vi "File Rollover.vi"() -> ()   [LabVIEW 2018]
uses:
  src/api/logger_class/Log Levels.ctl
  src/api/configuration/handlers/file_handler/File Handler.lvclass
  C:/Users/Colin/Documents/software_projects/labview/glog/src/api/extension/formatting_handler_interface/Formatting Handler.lvclass
  src/api/logger_class/Log (Parts).vi
  src/api/logger_class/Logger.lvclass
panel:
  in  "delete when done?":bool=TRUE
  out "error out":errorcluster
  out "2 files? (post-rollover)":bool
  out "1 file? (2nd)":bool
  out "1 file? (1st)":bool
  # "Locals"
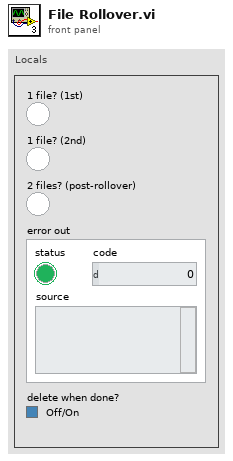
[diagram p1: front panel]
types:
  T1 = typedef "GLog.lvlib/Logger.lvclass/Log Levels.ctl" = enum16{"Trace", "Debug", "Info", "Warning", "Error", "Critical"}
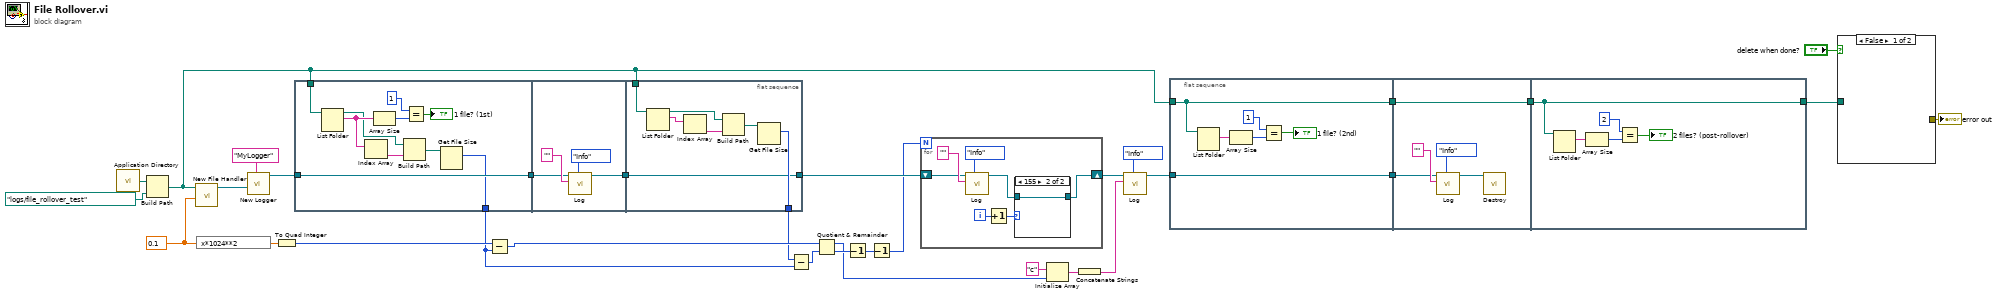
[diagram p0: block diagram]
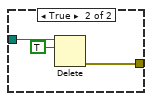
[diagram p3: hidden frame]
diagram:
  w26 = 0.1 ("rollover threshold [MB](50)")
  n1 = call <vilib>:"Application Directory.vi"() -> ("Application Directory"=w30:path)
  n2 = Build Path(base path=w30, name or relative path=path "logs/file_rollover_test") -> (appended path=w7:path)
  n3 = call "New File Handler.vi"("max file size [MB](50)"=w26, "log directory (<app dir>/logs)"=w7) -> ("file handler"=w31:refnum<class "File Handler.lvclass">)  [unwired: 9 in]
  n4 = expression code="x*1024**2"(w26) -> (w14:dbl)
  n5 = call "New Logger.vi"("name (\"Default\")"="MyLogger" ("name"), "log handler (file handler)"=w31) -> ("logger"=w9:refnum<class "Logger.lvclass">)  [unwired: 8 in, 1 out]
  n6 = To Quad Integer(1:w14) -> (0:w6:i64)
  n7 = flat-sequence {
    tunnel: w9 -> [w42]
    tunnel: [w42] -> w8
    tunnel: w7 -> [w35]
    tunnel: [w33] -> w4
    tunnel: [w43] -> w10
    tunnel: w8 -> [w44]
    tunnel: [w50] -> w3
    tunnel: w7 -> [w49]
    tunnel: [w48] -> w17
    tunnel: w10 -> [w48]
    frame #0 {
      n8 = List Folder(path=w35) -> (path out=w37:path, filenames=w39:string[])  [unwired: 3 in, 2 out]
      n9 = Index Array(array=w39) -> (element=w38:string)  [unwired: 1 in]
      n10 = Array Size(array=w39) -> (size(s)=w40:i32)
      n11 = Build Path(base path=w37, name or relative path=w38) -> (appended path=w36:path)
      n12 = Equal?(x=1, y=w40) -> (x = y?=→"1 file? (1st)":bool)
      n13 = Get File Size(file=w36) -> (size (in bytes)=w33:i64)  [unwired: 1 in, 2 out]
    }
    frame #1 {
      n14 = call-poly "Log.vi"("log level"=Log_Levels."Info" ("level"), "message"="", "logger in"=w44) -> ("logger out"=w43:refnum<class "Logger.lvclass">)  [unwired: 8 in]
    }
    frame #2 {
      n15 = List Folder(path=w49) -> (path out=w51:path, filenames=w53:string[])  [unwired: 3 in, 2 out]
      n16 = Index Array(array=w53) -> (element=w52:string)  [unwired: 1 in]
      n17 = Build Path(base path=w51, name or relative path=w52) -> (appended path=w47:path)
      n18 = Get File Size(file=w47) -> (size (in bytes)=w50:i64)  [unwired: 1 in, 2 out]
    }
  }
  n19 = Subtract(x=w6, y=w4) -> (x-y=w5:i64)
  n20 = Subtract(x=w3, y=w4) -> (x-y=w2:i64)
  n21 = Quotient & Remainder(x=w5, y=w2) -> (x-y*floor(x/y)=w19:i64, floor(x/y)=w25:i64)
  n22 = Decrement(x=w25) -> (x-1=w24:i64)
  n23 = Decrement(x=w24) -> (x-1=w16:i64)
  n24 = for {
    N: w16 -> [_]
    shift-right: [w55] -> w23
    shift-left: w17 -> [w57]
    i -> [w58]
    n25 = call-poly "Log.vi"("log level"=Log_Levels."Info" ("level"), "message"="", "logger in"=w57) -> ("logger out"=w56:refnum<class "Logger.lvclass">)  [unwired: 8 in]
    n26 = Increment(x=w58) -> (x+1=w54:i32)
    n27 = case shown="155" w54 {
      tunnel: w56 -> [w61 w62]
      tunnel: [w61 w62] -> w55
      frame Default {
      }
      frame 155 {
      }
    }
  }
  n28 = Initialize Array("c" ("message"), w19) -> (w21:string[])
  n29 = Concatenate Strings(w21) -> (w18:string)
  n30 = call-poly "Log.vi"("log level"=Log_Levels."Info" ("level"), "message"=w18, "logger in"=w23) -> ("logger out"=w12:refnum<class "Logger.lvclass">)  [unwired: 8 in]
  n31 = flat-sequence {
    tunnel: w7 -> [w64]
    tunnel: w12 -> [w65]
    tunnel: [w65] -> w29
    tunnel: [w64] -> w28
    tunnel: w29 -> [w70]
    tunnel: w28 -> [w73]
    tunnel: [w73] -> w27
    tunnel: w27 -> [w75]
    tunnel: [w75] -> w15
    frame #0 {
      n32 = List Folder(path=w64) -> (filenames=w68:string[])  [unwired: 3 in, 3 out]
      n33 = Array Size(array=w68) -> (size(s)=w67:i32)
      n34 = Equal?(x=1, y=w67) -> (x = y?=→"1 file? (2nd)":bool)
    }
    frame #1 {
      n35 = call-poly "Log.vi"("log level"=Log_Levels."Info" ("level"), "message"="", "logger in"=w70) -> ("logger out"=w69:refnum<class "Logger.lvclass">)  [unwired: 8 in]
      n36 = call "Destroy.vi"("logger in"=w69) -> ()  [unwired: 9 in, 2 out]
    }
    frame #2 {
      n37 = List Folder(path=w75) -> (filenames=w78:string[])  [unwired: 3 in, 3 out]
      n38 = Array Size(array=w78) -> (size(s)=w77:i32)
      n39 = Equal?(x=2, y=w77) -> (x = y?=→"2 files? (post-rollover)":bool)
    }
  }
  n40 = case shown="False" "delete when done?" {
    tunnel: w15 -> [_ w80]
    tunnel: [_ w79] -> w13
    frame False {
    }
    frame True {
      n41 = Delete(path (use dialog)=w80, entire hierarchy (F)=TRUE) -> (error out=w79:errorcluster)  [unwired: 3 in, 2 out]
    }
  }
  "error out" <- w13
